vi "ep_Compute Third Current (Vectors).vi"(0 "one period fundamental current vectors in":T2(array[cluster]), 5 "wiring":T3, 11 "error in (no error)":errorcluster) -> (4 "one period fundamental current vectors out":T2(array[cluster]), 15 "error out":errorcluster)   [LabVIEW 2011, in "NI_EP_Power Quality.lvlib"]
uses:
  <vilib>/addons/Electrical Power/PQ/NI_EP_Power Quality.lvlib
  <vilib>/addons/Electrical Power/PQ/Common/Controls/ep_AI Data Channel.ctl
  <vilib>/addons/Electrical Power/PQ/Common/Controls/ep_Wiring.ctl
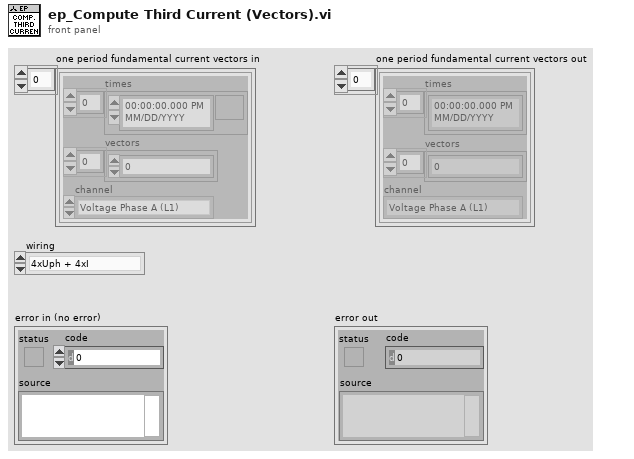
[diagram p1: front panel]
types:
  T1 = typedef "NI_EP_Power Quality.lvlib/ep_AI Data Channel.ctl" = enum16{"Voltage Phase A (L1)", "Voltage Phase B (L2)", "Voltage Phase C (L3)", "Voltage Phase N (Neutral)", "Current Phase A (L1)", "Current Phase B (L2)", "Current Phase C (L3)", "Current Phase N (Neutral)"}
  T2 = cluster{"times":timestamp[], "vectors":cdb[], "channel":T1}[]
  T3 = typedef "NI_EP_Power Quality.lvlib/ep_Wiring.ctl" = enum16{"4xUph + 4xI", "3xUph + 4xI", "3xUline + 4xI", "3xUph + 3xI", "3xUline + 3xI", "3xUph + 2xI", "3xUline + 2xI", "1xUph + 1xI"}
  T4 = cluster{"times":timestamp[], "vectors":cdb[], "channel":T1}
  T5 = cluster{"times":timestamp[], cdb[], "AI data channel":T1}
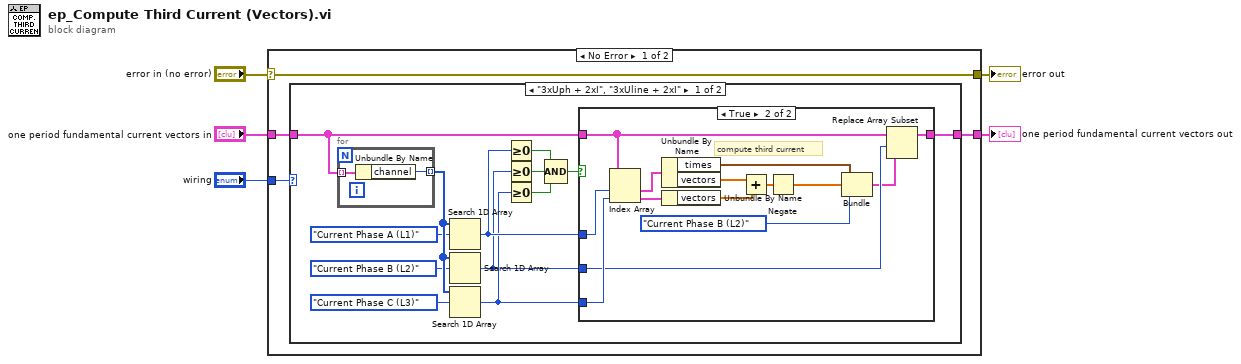
[diagram p0: block diagram]
diagram:
  n1 = case shown="No Error" "error in (no error)" {
    selector: "error in (no error)" -> [w6 w41]
    tunnel: "wiring" -> [w9 _]
    tunnel: [w8 _] -> w4
    tunnel: "one period fundamental current vectors in" -> [w7 _]
    tunnel: [w6 w41] -> w1
    frame No Error {
      n2 = case shown="\"3xUph + 2xI\", \"3xUline + 2xI\"" w9 {
        tunnel: w7 -> [w11 w40]
        tunnel: [w22 w40] -> w8
        frame "3xUph + 2xI", "3xUline + 2xI" {
          n3 = for {
            tunnel: w11 -> [w39] mode=indexing
            tunnel: [w38] -> w19 mode=indexing
            n4 = Unbundle By Name(w39) -> ("channel"=w38:T1)
          }
          n5 = Search 1D Array(1D array=w19, element=ep_AI_Data_Channel."Current Phase A (L1)" ("AI data channel")) -> (index of element=w14:i32)  [unwired: 1 in]
          n6 = Search 1D Array(1D array=w19, element=ep_AI_Data_Channel."Current Phase B (L2)" ("AI data channel")) -> (index of element=w12:i32)  [unwired: 1 in]
          n7 = Search 1D Array(1D array=w19, element=ep_AI_Data_Channel."Current Phase C (L3)" ("AI data channel")) -> (index of element=w13:i32)  [unwired: 1 in]
          n8 = Greater Or Equal To 0?(x=w14) -> (x >= 0?=w10:bool)
          n9 = Greater Or Equal To 0?(x=w12) -> (x >= 0?=w20:bool)
          n10 = Greater Or Equal To 0?(x=w13) -> (x >= 0?=w21:bool)
          n11 = Compound Arithmetic op=AND(w10, w20, w21) -> (w15:bool)
          n12 = case shown="True" w15 {
            tunnel: [w23 w37] -> w22
            tunnel: w11 -> [w23 w36]
            tunnel: w14 -> [_ w35]
            tunnel: w13 -> [_ w34]
            tunnel: w12 -> [_ w33]
            frame False {
            }
            frame True {
              # "compute third current"
              n13 = Index Array(array=w36, index #1=w35, index #2=w34) -> (element #1=w32:T4, element #2=w31:T4)
              n14 = Unbundle By Name(w32) -> ("times"=w27:timestamp[], "vectors"=w29:cdb[])
              n15 = Unbundle By Name(w31) -> ("vectors"=w30:cdb[])
              n16 = Add(x=w29, y=w30) -> (x+y=w28:cdb[])
              n17 = Negate(x=w28) -> (-x=w26:cdb[])
              n18 = Bundle("times"=w27, w26, "AI data channel"=ep_AI_Data_Channel."Current Phase B (L2)") -> (w24:T5)  [unwired: 1 in]
              n19 = Replace Array Subset(array=w36, new element=w24, index=w33) -> (w37:T2)
            }
          }
        }
        frame Default {
        }
      }
    }
    frame Error {
    }
  }
  "error out" <- w1
  "one period fundamental current vectors out" <- w4
